vi "Get Channel Settings (Array).vi"(1 "Channel Settings typedef":T1[](array[typedef])) -> (0 "Channel Settings ducktype":T4(array[cluster]))   [LabVIEW 2021, in "Settings.lvlib"]
uses:
  Acquisition/Channel Settings.ctl
  Settings.lvlib
  Acquisition/IO Device.ctl
  Acquisition/Acquisition.lvlib
  Acquisition/Sensor Type.ctl
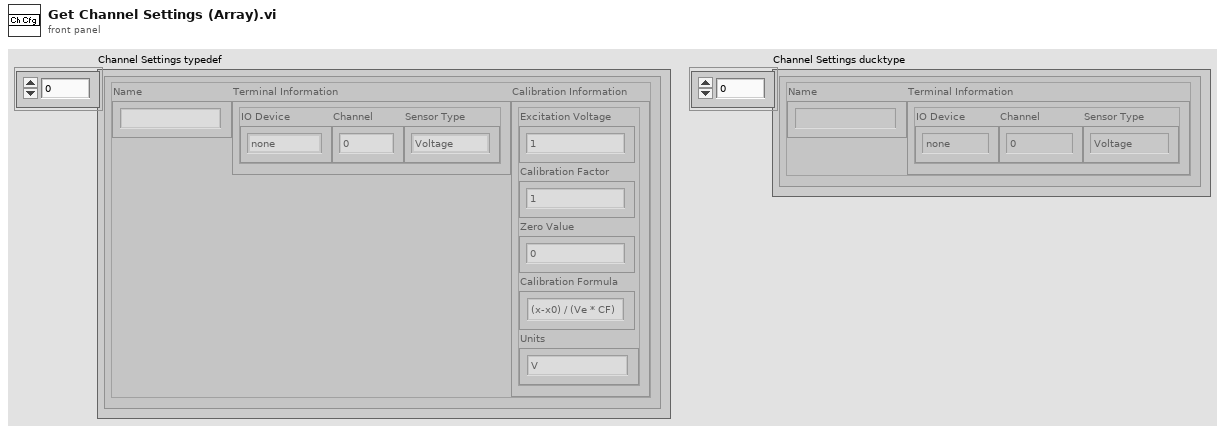
[diagram p1: front panel]
types:
  T1 = typedef "Acquisition.lvlib/Channel Settings.ctl" = cluster{"Name":string, "Terminal Information":cluster{"IO Device":T2, "Channel":i32, "Sensor Type":T3}, "Calibration Information":cluster{"Excitation Voltage":dbl, "Calibration Factor":dbl, "Zero Value":dbl, "Calibration Formula":string, "Units":string}}
  T2 = typedef "Acquisition.lvlib/IO Device.ctl" = enum16{"none", "9219", "9401"}
  T3 = typedef "Acquisition.lvlib/Sensor Type.ctl" = enum16{"Voltage", "Load", "Pressure", "Encoder"}
  T4 = cluster{"Name":string, "Terminal Information":cluster{"IO Device":T2, "Channel":i32, "Sensor Type":T3}}[]
  T5 = cluster{"Name":string, "Terminal Information":cluster{"IO Device":T2, "Channel":i32, "Sensor Type":T3}}
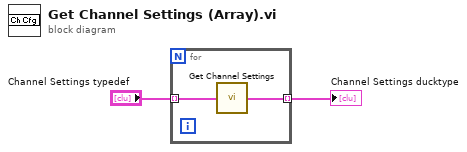
[diagram p0: block diagram]
diagram:
  n1 = for {
    tunnel: "Channel Settings typedef" -> [w4] mode=indexing
    tunnel: [w3] -> w1 mode=indexing
    n2 = call "Get Channel Settings.vi"("Channel Settings typedef"=w4) -> ("Channel Settings ducktype"=w3:T5)
  }
  "Channel Settings ducktype" <- w1
